vi "UpData.vi"(6 "TableName":string, 8 "error in (no error)":errorcluster caption="错误输入（无错误）", 9 "TestValue":T1, 10 "SerialNumber":string, 11 "DataBase in":refnum<class "DataBase.lvclass">) -> (0 "error out":errorcluster caption="错误输出", 3 "DataBase out":refnum<class "DataBase.lvclass">)   [LabVIEW 2019, in "DataBase.lvlib" / "DataBase.lvclass"]
uses:
  DataBase.lvclass
  DataBase.lvclass/DataBase.ctl
  <vilib>/addons/database/NI_Database_API.lvlib
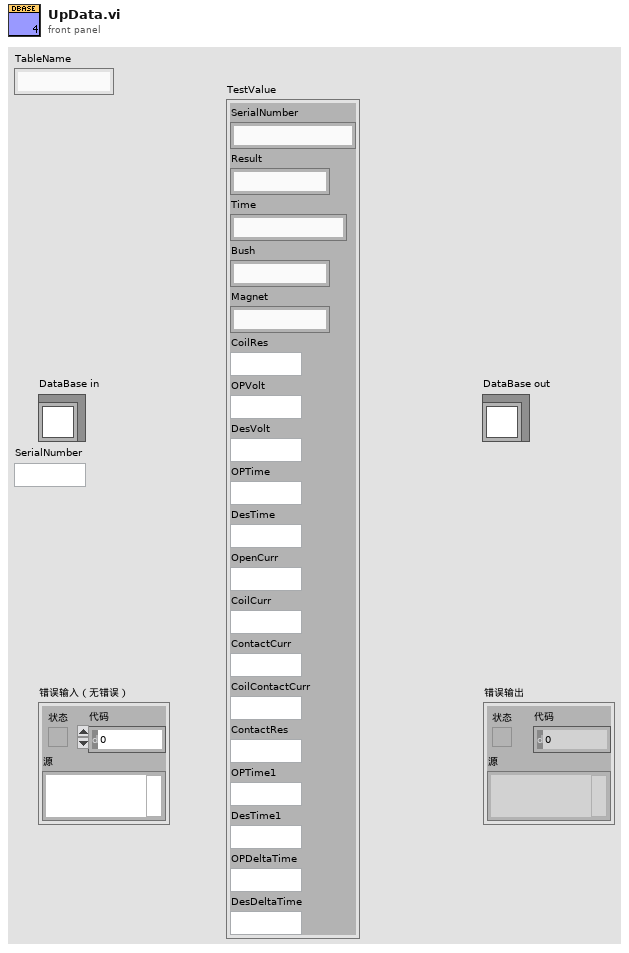
[diagram p1: front panel]
types:
  T1 = cluster{"SerialNumber":string, "Result":string, "Time":string, "Bush":string, "Magnet":string, "CoilRes":string, "OPVolt":string, "DesVolt":string, "OPTime":string, "DesTime":string, "OpenCurr":string, "CoilCurr":string, "ContactCurr":string, "CoilContactCurr":string, "ContactRes":string, "OPTime1":string, "DesTime1":string, "OPDeltaTime":string, "DesDeltaTime":string}
  T2 = typedef "NI_Database_API.lvlib/Conn ObjectReference.ctl" = refnum<k1>
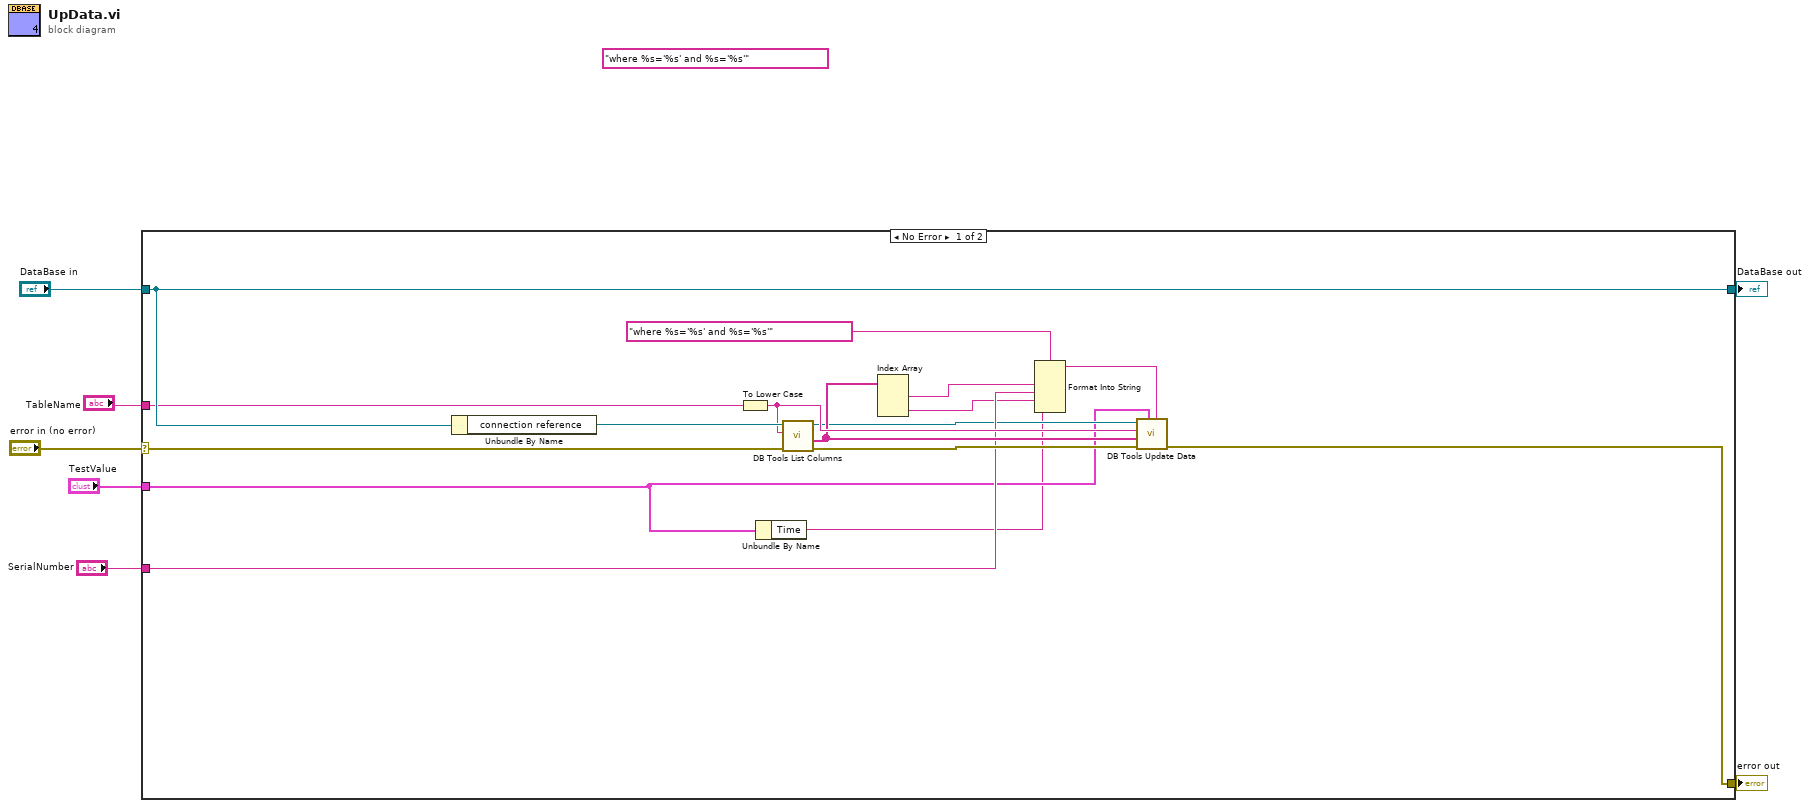
[diagram p0: block diagram]
diagram:
  (unwired) "where %s='%s' and %s='%s'" ("format string")
  n1 = case shown="No Error" "error in (no error)" {
    selector: "error in (no error)" -> [w19 w25]
    tunnel: [w18 w25] -> w6
    tunnel: [w20 w24] -> w4
    tunnel: "DataBase in" -> [w20 w24]
    tunnel: "SerialNumber" -> [w14 _]
    tunnel: "TestValue" -> [w10 _]
    tunnel: "TableName" -> [w8 _]
    frame No Error {
      n2 = Unbundle By Name(w20) -> ("connection reference"=w22:T2)
      n3 = To Lower Case(string=w8) -> (all lower case string=w17:string)
      n4 = Unbundle By Name(w10) -> ("Time"=w9:string)
      n5 = call <vilib>:"DB Tools List Columns.vi"("error in (no error)"=w19, "table"=w17, "connection reference"=w22) -> ("error out"=w23:errorcluster, "columns"=w16:string[], "connection reference out"=w12:T2)  [unwired: 1 in, 1 out]
      n6 = Index Array(array=w16) -> (element #1=w15:string, element #3=w11:string)  [unwired: 3 in, 1 out]
      n7 = Format Into String(format string="where %s='%s' and %s='%s'", w15, w14, w11, w9) -> (resulting string=w13:string)  [unwired: 2 in, 1 out]
      n8 = call <vilib>:"DB Tools Update Data.vi"("condition"=w13, "data"=w10, "error in (no error)"=w23, "columns"=w16, "table"=w17, "connection reference"=w12) -> ("error out"=w18:errorcluster)  [unwired: 4 in, 1 out]
    }
    frame Error {
    }
  }
  "error out" <- w6
  "DataBase out" <- w4
